vi "Check_TRF_TSP Check.vi"(8 "error in":errorcluster, 10 "TRF Cluster":T1, 11 "TSP Cluster":T2) -> (0 "error out":errorcluster)   [LabVIEW 2012]
doc: "This .vi prompts the user to select at least one of TRF or TSP boolean if neither have been selected."
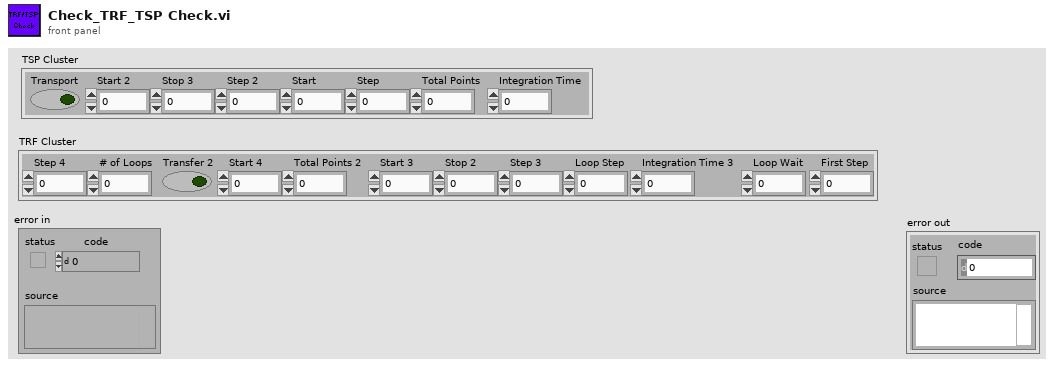
[diagram p1: front panel]
types:
  T1 = cluster{"Step 4":dbl, "# of Loops":dbl, "Transfer 2":bool, "Start 4":dbl, "Total Points 2":u16, "Start 3":dbl, "Stop 2":dbl, "Step 3":dbl, "Loop Step":dbl, "Integration Time 3":u32, "Loop Wait":dbl, "First Step":dbl}
  T2 = cluster{"Transport":bool, "Start 2":dbl, "Stop 3":dbl, "Step 2":dbl, "Start":dbl, "Step":dbl, "Total Points":u16, "Integration Time":u32}
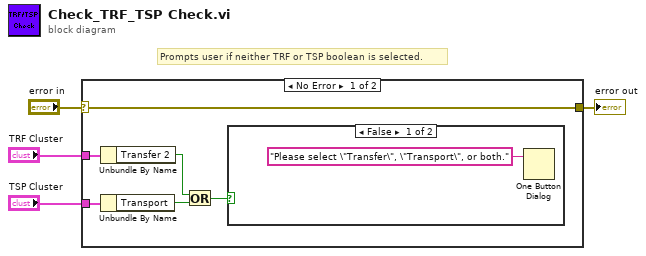
[diagram p0: block diagram]
diagram:
  # "Prompts user if neither TRF or TSP boolean is selected."
  n1 = case shown="No Error" "error in" {
    selector: "error in" -> [w7 w12]
    tunnel: [w7 w12] -> w3
    tunnel: "TRF Cluster" -> [w6 _]
    tunnel: "TSP Cluster" -> [w5 _]
    frame No Error {
      n2 = Unbundle By Name(w6) -> ("Transfer 2"=w9:bool)
      n3 = Unbundle By Name(w5) -> ("Transport"=w10:bool)
      n4 = Or(x=w9, y=w10) -> (x .or. y?=w8:bool)
      n5 = case shown="False" w8 {
        frame False {
          n6 = One Button Dialog(message="Please select \"Transfer\", \"Transport\", or both.") -> ()  [unwired: 1 in, 1 out]
        }
        frame True {
        }
      }
    }
    frame Error {
    }
  }
  "error out" <- w3
